vi "Get Collatz sequence-with array output-v2.vi"(8 "error in (no error)":errorcluster, 11 "n":i32) -> (0 "error out":errorcluster, 2 "no. of elements (chain length)":i32, 3 "Collatz sequence of n":i32[](array[numeric]))   [LabVIEW 2021, in "Numeric Utilities.lvlib"]
doc: "Warning: This VI runs out of memory for some values of n."
uses:
  Numeric Utilities.lvlib
panel:
  in  "Dev: stop early":bool
  out "iteration":i32
  # "Development\ncontrols/indicators useful for development and testing, but which are not outputs of the VI"
  # "Input\nInputs to the VI"
  # "Output\nOutputs of the VI"
  # "Description\n\nWarning: This VI runs out of memory for some values of n."
  # "113,383"
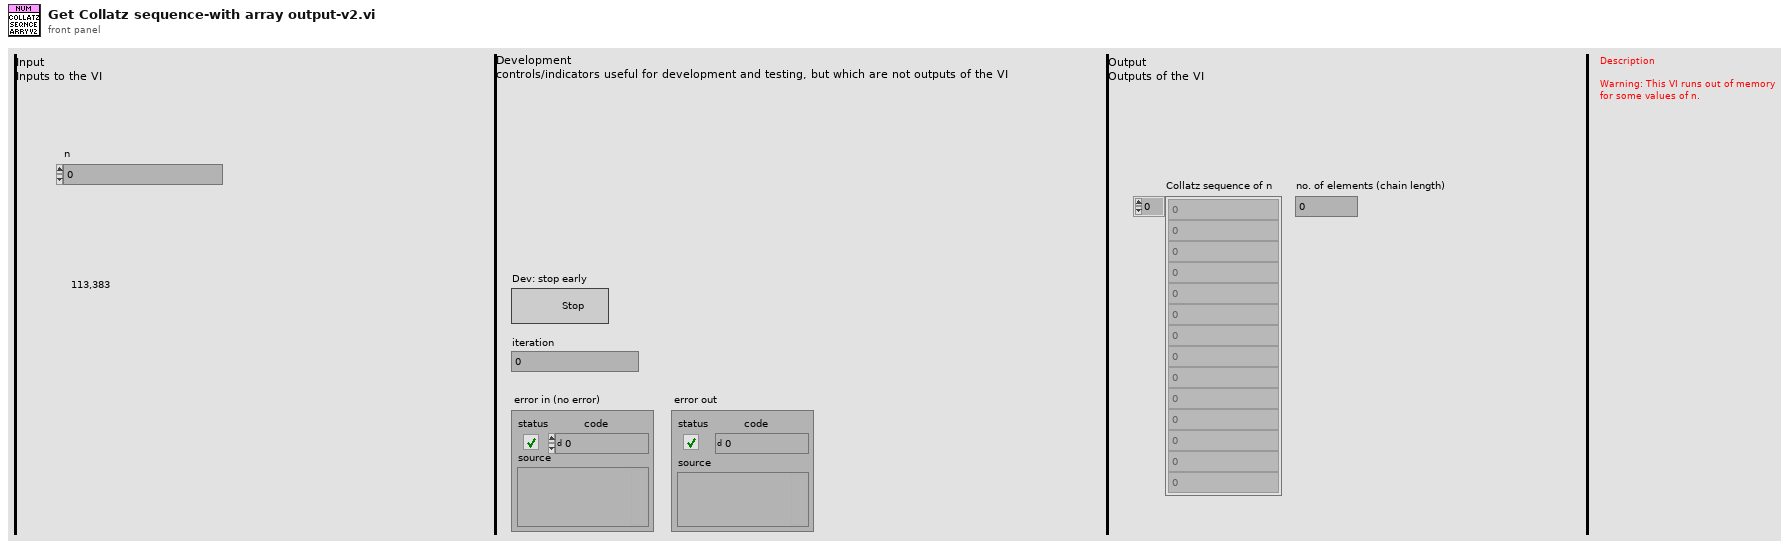
[diagram p1: front panel]
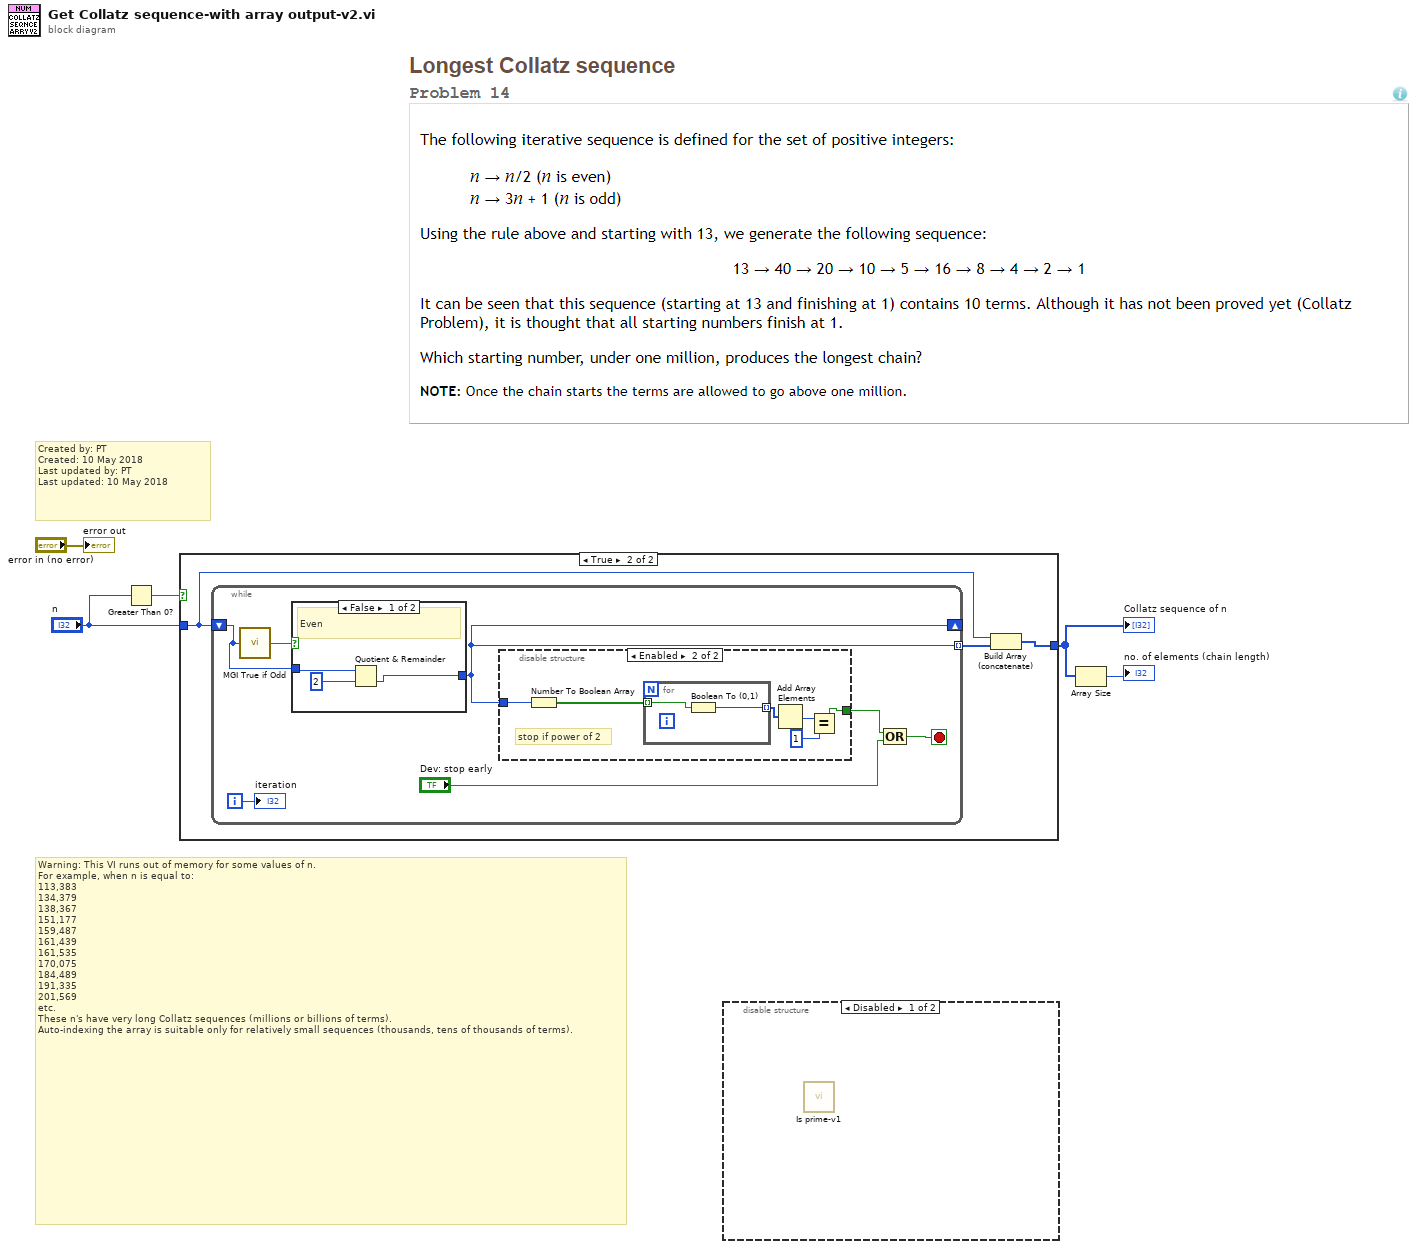
[diagram p0: block diagram]
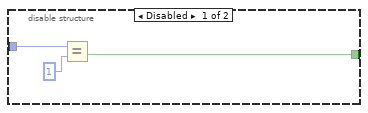
[diagram p4: hidden frame]
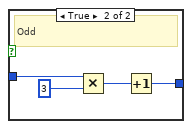
[diagram p5: hidden frame]
diagram:
  # "Warning: This VI runs out of memory for some values of n. \nFor example, when n is equal to:\n113,383\n134,379\n138,367\n151,177\n159,487\n161,439\n161,535\n170,075\n184,489\n191,335\n201,569\netc.\nThese n's have very long Collatz sequences (millions or billions of terms). \nAuto-indexing the array is suitable only for relatively small sequences (thousands, tens of thousands of terms)."
  # "Created by: PT\nCreated: 10 May 2018\nLast updated by: PT\nLast updated: 10 May 2018"
  n1 = Greater Than 0?(x="n") -> (x > 0?=w4:bool)
  n2 = case shown="True" w4 {
    tunnel: "n" -> [_ w6]
    tunnel: [_ w7] -> w2
    frame False {
    }
    frame True {
      n3 = while {
        shift-right: [w9] -> _
        shift-left: w6 -> [w14]
        tunnel: [w9] -> w8 mode=indexing
        i -> [w13]
        stop <- w11 stop-if-true
        n4 = call <userlib>:"MGI True if Odd.vi"("Integer"=w14) -> ("Odd?"=w15:bool)
        n5 = case shown="False" w15 {
          tunnel: w14 -> [w29 w33]
          tunnel: [w27 w30] -> w9
          frame False {
            # "Even"
            n6 = Quotient & Remainder(x=w29, y=2) -> (floor(x/y)=w27:i32)  [unwired: 1 out]
          }
          frame True {
            # "Odd"
            n7 = Multiply(x=w33, y=3) -> (x*y=w31:i32)
            n8 = Increment(x=w31) -> (x+1=w30:i32)
          }
        }
        n9 = disable-structure shown="Enabled" {
          disable-tunnel: [w17 w19] -> w12
          disable-tunnel: w9 -> [w16 w24]
          frame Disabled {
            n10 = Equal?(x=w16, y=1) -> (x = y?=w17:bool)
          }
          frame Enabled {
            # "stop if power of 2"
            n11 = Number To Boolean Array(number=w24) -> (Boolean array=w23:bool[])
            n12 = for {
              tunnel: w23 -> [w26] mode=indexing
              tunnel: [w25] -> w22 mode=indexing
              n13 = Boolean To (0,1)(Boolean=w26) -> (0, 1=w25:i16)
            }
            n14 = Add Array Elements(numeric array=w22) -> (sum=w21:i16)
            n15 = Equal?(x=w21, y=i16 1) -> (x = y?=w19:bool)
          }
        }
        n16 = Compound Arithmetic op=OR(w12, "Dev: stop early") -> (w11:bool)
        "iteration" <- w13
      }
      n17 = Build Array (concatenate)(w6, w8) -> (w7:i32[])
    }
  }
  "Collatz sequence of n" <- w2
  n18 = disable-structure shown="Disabled" {
    frame Disabled {
      n19 = call "Is prime-v1.vi"() -> ()  [unwired: 9 in, 3 out]
    }
    frame Enabled {
    }
  }
  n20 = Array Size(array=w2) -> (size(s)=→"no. of elements (chain length)":i32)
  "error out" <- "error in (no error)"
